vi "ConvertHeaterDisplayStateToCSVString.vi"(11 "Heater Display State":T1) -> (3 "CSV String":string)   [LabVIEW 2012]
uses:
  HeaterDisplayState.ctl
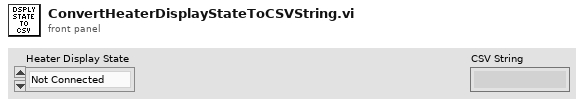
[diagram p1: front panel]
types:
  T1 = typedef "HeaterDisplayState.ctl" = enum16{"Not Connected", "Run", "Standby"}
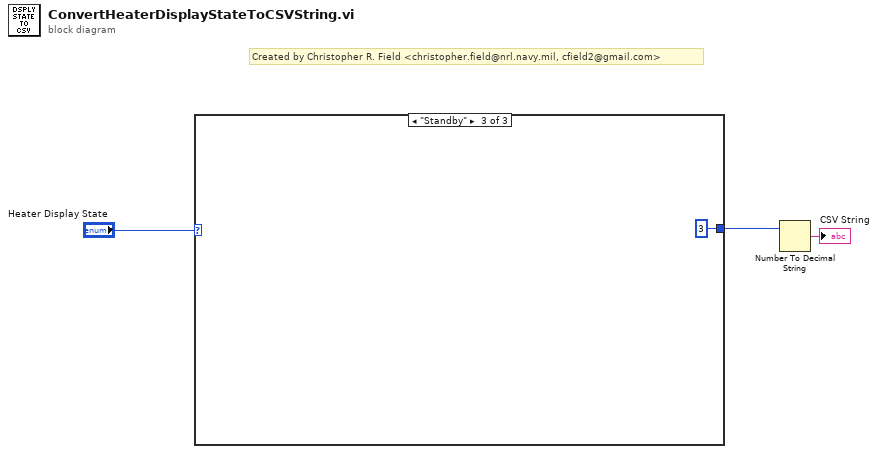
[diagram p0: block diagram]
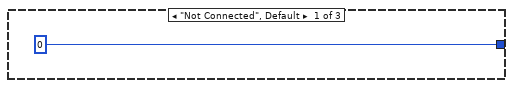
[diagram p2: hidden frame]
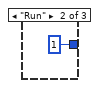
[diagram p3: hidden frame]
diagram:
  # "Created by Christopher R. Field <christopher.field@nrl.navy.mil, cfield2@gmail.com>"
  n1 = case shown="\"Standby\"" "Heater Display State" {
    tunnel: [0 1 3] -> w2
    frame "Not Connected", Default {
    }
    frame "Run" {
    }
    frame "Standby" {
    }
  }
  n2 = Number To Decimal String(number=w2) -> (decimal integer string=→"CSV String":string)  [unwired: 1 in]
